vi "Init.vi"(8 "error in (no error)":errorcluster, 11 "BCReg":refnum<data-value>) -> (0 "error out":errorcluster, 3 "BCReg":refnum<data-value>)   [LabVIEW 2014, in "BusController.lvlib" / "BCReg.lvclass"]
uses:
  BCReg.lvclass
  BCReg.lvclass/BCReg.ctl
  Accessors/Write Reg.vi
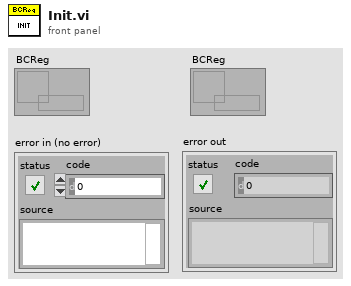
[diagram p1: front panel]
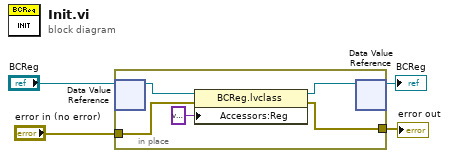
[diagram p0: block diagram]
diagram:
  n1 = in-place {
    in-place-border: "error in (no error)" -> [w8]
    in-place-border: [w5] -> w1
    n2 = in-place-dvr #1("BCReg") -> (w9:refnum<class "BCReg.lvclass">)  [unwired: 1 out]
    n3 = property class="BCReg.lvclass"(reference=w9, error in=w8, "Accessors:Reg"=variant ("Reg")) -> (reference out=w6:refnum<class "BCReg.lvclass">, error out=w5:errorcluster)
    n4 = in-place-dvr #1(w6) -> (→"BCReg":refnum<data-value>)  [unwired: 1 out]
  }
  "error out" <- w1
